vi "goto.vi"(0 "连接ID":refnum<k5>, 1 "x":dbl, 2 "y":dbl, 3 "z":dbl, 4 "v":dbl=10.0) -> (5 "连接ID":refnum<k5>)   [LabVIEW 2017]
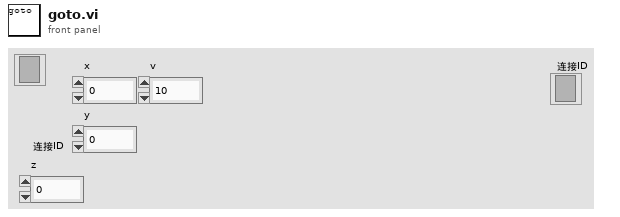
[diagram p1: front panel]
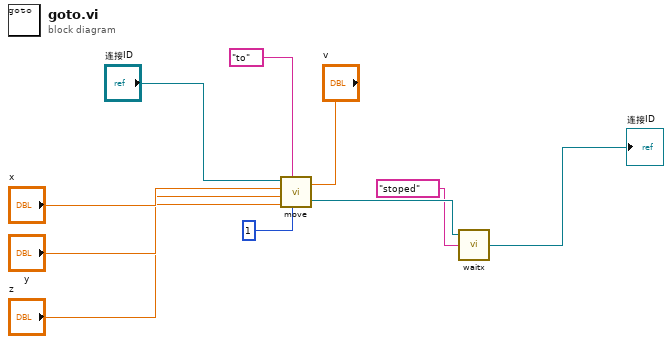
[diagram p0: block diagram]
diagram:
  n1 = call "move.vi"("v"="v", "n"=1, "String"="to", "z"="z", "y"="y", "x"="x", "连接ID"="连接ID") -> ("连接ID输出"=w4:refnum<k5>)
  n2 = call "waitx.vi"("String Value"="stoped", "连接ID"=w4) -> ("连接ID 2"=→"连接ID":refnum<k5>)  [unwired: 1 in]
